vi "Remove_Spaces.vi"(5 "input string":string) -> (2 "result string":string)   [LabVIEW 2021]
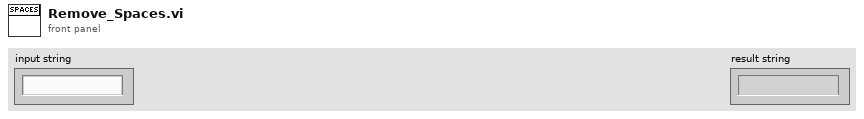
[diagram p1: front panel]
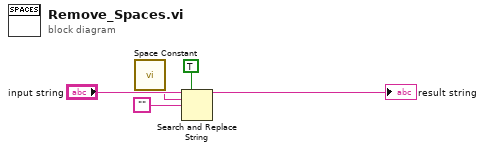
[diagram p0: block diagram]
diagram:
  n1 = call <vilib>:"Space Constant.vi"() -> ("String"=w3:string)
  n2 = Search and Replace String(replace all?=TRUE ("replace all? (F)"), input string="input string", search string=w3, replace string="") -> (result string=→"result string":string)  [unwired: 4 in, 3 out]
